vi "Cleanup.vi"(8 "error in (no error)":errorcluster, 11 "Ambient Light Bricklet in":refnum<class "Temperature IR Bricklet.lvclass">) -> (0 "error out":errorcluster)   [LabVIEW 2011, in "Tinkerforge.lvlib" / "Temperature IR Bricklet.lvclass"]
doc: "This VI is the child implementation of \"Cleanup.vi\" and releases all synchronization objects of this child object."
uses:
  Temperature IR Bricklet.lvclass
  Temperature IR Bricklet.lvclass/Temperature IR Bricklet.ctl
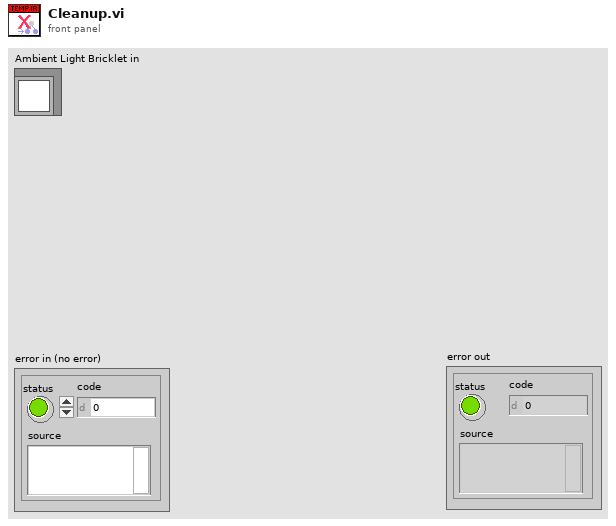
[diagram p1: front panel]
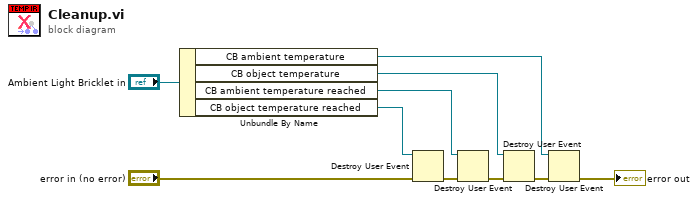
[diagram p0: block diagram]
diagram:
  n1 = Unbundle By Name("Ambient Light Bricklet in") -> ("CB ambient temperature"=w1:refnum<user-event>, "CB object temperature"=w2:refnum<user-event>, "CB ambient temperature reached"=w6:refnum<user-event>, "CB object temperature reached"=w8:refnum<user-event>)
  n2 = Destroy User Event(user event=w8, error in="error in (no error)") -> (error out=w7:errorcluster)
  n3 = Destroy User Event(user event=w6, error in=w7) -> (error out=w5:errorcluster)
  n4 = Destroy User Event(user event=w2, error in=w5) -> (error out=w3:errorcluster)
  n5 = Destroy User Event(user event=w1, error in=w3) -> (error out=→"error out":errorcluster)
